vi "DpcGetReg.vi"(8 "Error In":errorcluster, 10 "Register Address":u8, 11 "Device Handle":u32) -> (0 "Error Out":errorcluster, 1 "Task ID":u16, 2 "Data":u8, 3 "Device Handle":u32)   [LabVIEW 2011, in "LVH-Adept.lvlib" / "DPCUTIL.lvlib"]
uses:
  DPCUTIL.lvlib
  Private/Type Defs/Error.ctl
  dpcutil.dll
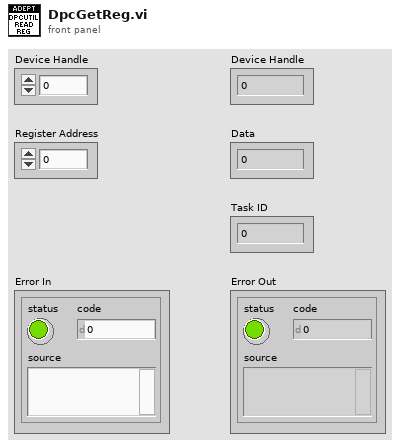
[diagram p1: front panel]
types:
  T1 = typedef "LVH-Adept.lvlib/DPCUTIL.lvlib/Error.ctl" = enum16{"Unknown", "Open Data", "Wait For Transaction", "Put Reg", "Get Reg", "Close Data"}
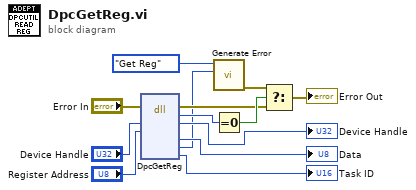
[diagram p0: block diagram]
diagram:
  n1 = dll-call lib="dpcutil.*" fn="DpcGetReg"(error in="Error In", "hif"="Device Handle", "bAddr"="Register Address") -> (error out=w3:errorcluster, "return type"=w4:i32, "hif"=→"Device Handle":u32, "pbData"=→"Data":u8, "perc"=w1:i32, "ptrid"=→"Task ID":u16)  [unwired: 6 in, 1 out]
  n2 = call "Generate Error.vi"("Adept Error Code"=w1, "DPCUTIL Error"=Error."Get Reg") -> ("Error Out"=w7:errorcluster)  [unwired: 9 in]
  n3 = Equal To 0?(x=w4) -> (x = 0?=w6:bool)
  n4 = Select(t=w7, s=w6, f=w3) -> (s? t:f=→"Error Out":errorcluster)
